vi "RP Read RX FIFO.vi"(6 "FIFO Bytes per read":i32=49152, 8 "Error In":errorcluster, 11 "connection ID":refnum<k5>) -> (0 "Error Out":errorcluster, 1 "Y":i32[](array[numeric]), 2 "X":i32[](array[numeric]), 3 "connection ID out":refnum<k5>, 4 "F":i32[](array[numeric]))   [LabVIEW 2015]
uses:
  RP Command.ctl
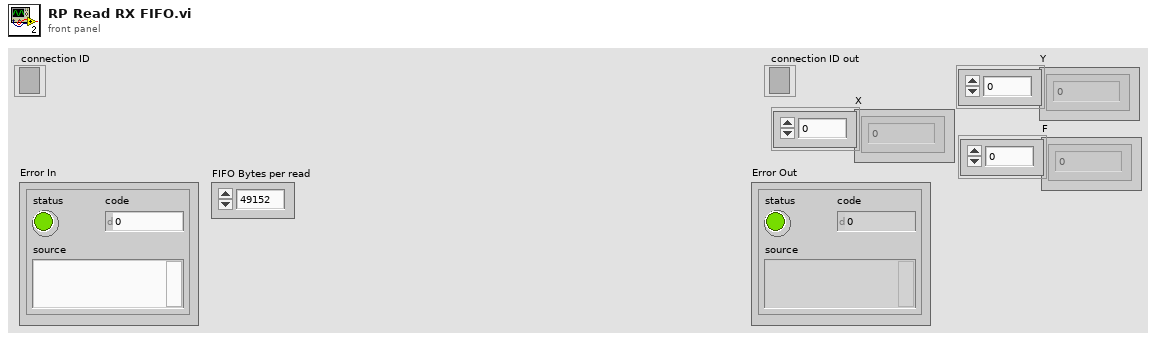
[diagram p1: front panel]
types:
  T1 = enum16{"big-endian, network order", "native, host order", "little-endian"}
  T2 = typedef "RP Command.ctl" = enum16{"Set frequency", "Arm and get data", "Stop server", "Get status", "Get temperature", "Set decimation", "Arm", "Software trigger", "Get whole buffer", "Get chunk", "System call", "Get config", "Set config", "Read FIFO"}
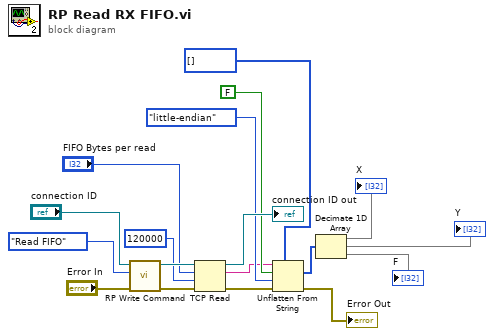
[diagram p0: block diagram]
diagram:
  n1 = call "RP Write Command.vi"("Error In"="Error In", "Command number"=RP_Command."Read FIFO", "connection ID"="connection ID") -> ("Error Out"=w16:errorcluster, "connection ID out"=w17:refnum<k5>)  [unwired: 6 in, 1 out]
  n2 = TCP Read(connection ID=w17, bytes to read="FIFO Bytes per read", error in (no error)=w16, 9:120000 ("timeout ms (25000)")) -> (connection ID out=→"connection ID out":refnum<k5>, data out=w6:string, error out=w5:errorcluster)  [unwired: 1 in]
  n3 = Unflatten From String(type=i32[] [], binary string=w6, data includes array or string size? (T)=FALSE, byte order (0:big-endian, network order)=T1."little-endian", error in (no error)=w5) -> (value=w7:i32[], error out=→"Error Out":errorcluster)  [unwired: 1 out]
  n4 = Decimate 1D Array(w7) -> (→"X":i32[], →"Y":i32[], →"F":i32[])
